vi "Update Case Item Result.vi"(9 "Status":T1, 10 "Test Case":string, 11 "Test Result Tree V2 in":refnum<class "Test Result Tree V2.lvclass">) -> (3 "Test Result Tree V2 out":refnum<class "Test Result Tree V2.lvclass">)   [LabVIEW 2020, in "Test Result Tree V2.lvclass"]
uses:
  Test Result Tree V2.lvclass
  Test Result Tree V2.lvclass/Test Result Tree V2.ctl
  Framework/Helper Classes/Test Tree/Test Tree.lvclass
  Utilities/LUnit Utilities.lvlib
  C:/Git/astemes-lunit/source/Framework/Helper Classes/Test Tree/Test Tree.lvclass
  C:/Git/astemes-lunit/source/Rewrite Project/Test Result Tree/Test Result Tree/Test Result Tree V2.lvclass
  C:/Git/astemes-lunit/source/Rewrite Project/Result Observer/Result Observer.lvclass
  Result/Status.ctl
  Result/Result.lvlib
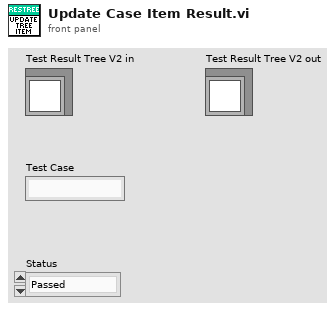
[diagram p1: front panel]
types:
  T1 = typedef "Result.lvlib/Status.ctl" = enum16{"Passed", "Failed", "Error", "Skipped", "Setup Error", "Broken", "Teardown Error"}
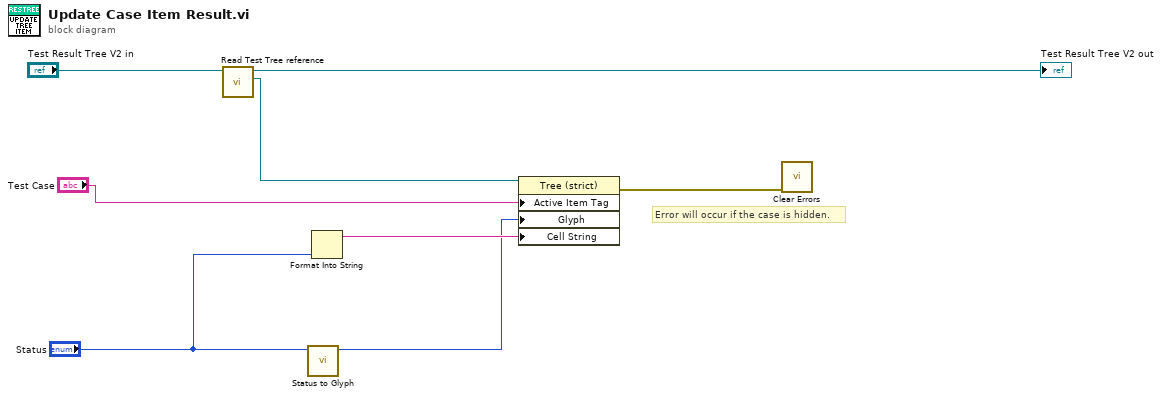
[diagram p0: block diagram]
diagram:
  # "Error will occur if the case is hidden."
  n1 = call "Read Test Tree reference.vi"("Test Tree in"="Test Result Tree V2 in") -> ("Test Tree reference"=w5:refnum<vi>, "Test Tree out"=→"Test Result Tree V2 out":refnum<class "Test Result Tree V2.lvclass">)  [unwired: 8 in, 1 out]
  n2 = call "Status to Glyph.vi"("Status"="Status") -> ("Listbox Symbol Ring Constant"=w1:i32)  [unwired: 10 in]
  n3 = Format Into String("Status") -> (resulting string=w2:string)  [unwired: 3 in, 1 out]
  n4 = property class="Tree (strict)"(reference=w5, "Active Item Tag"="Test Case", "Glyph"=w1, "Cell String"=w2) -> (error out=w8:errorcluster)  [unwired: 1 in, 1 out]
  n5 = call <vilib>:"Clear Errors.vi"("error in (no error)"=w8) -> ()  [unwired: 5 in, 2 out]
